vi "Read ELn Params.vi"(0 "Motor in":refnum<class "Motor.lvclass">, 11 "error in (no error)":errorcluster) -> (4 "Motor out":refnum<class "Motor.lvclass">, 6 "Limit- Enabled?":bool caption="Enabled?", 8 "Limit- Logic":enum16{"Low", "High"}(ring) caption="Logic", 10 "Limit- Mode":enum16{"Stop immediately", "Decelerate to Stop"}(ring) caption="Mode", 14 "Limit- Sensor ID":enum16{"N/A", "S1", "S2", "S3"}(ring), 15 "error out":errorcluster)   [LabVIEW 2016, in "Hardware.lvlib" / "Motor.lvlib" / "Motor.lvclass"]
uses:
  <userlib>/Common Components/Hardware/Motor/Motor/Motor.lvclass
  <userlib>/Common Components/Hardware/Motor/Motor/Motor.lvclass/Motor.ctl
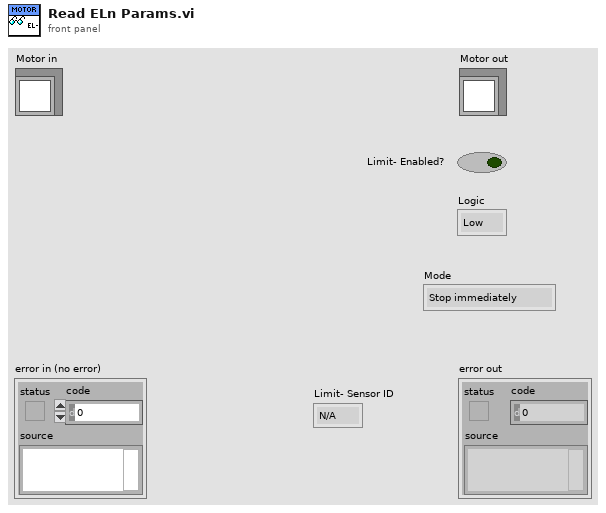
[diagram p1: front panel]
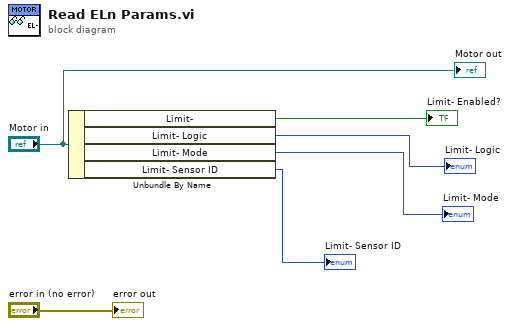
[diagram p0: block diagram]
diagram:
  n1 = Unbundle By Name("Motor in") -> ("Limit-"=→"Limit- Enabled?":bool, "Limit- Logic"=→"Limit- Logic":enum16{"Low", "High"}, "Limit- Mode"=→"Limit- Mode":enum16{"Stop immediately", "Decelerate to Stop"}, "Limit- Sensor ID"=→"Limit- Sensor ID":enum16{"N/A", "S1", "S2", "S3"})
  "error out" <- "error in (no error)"
  "Motor out" <- "Motor in"
